vi "Same.vi"() -> ()   [LabVIEW 2017, in "Assertions.Tests.lvlib" / "Assert Not Equal.lvlib"]
uses:
  Assert Not Equal.lvlib
  src/Transparent Assertions/Constraints/IsEqual/IsEqual.lvclass
  C:/Users/pasca/Projects/Home/TransparentAssertions/src/Transparent Assertions/Constraints/Constraint/Constraint.lvclass
  src/Transparent Assertions/Constraints/IsEqual/Create.vi
  src/Transparent Assertions/Constraints/LogicalNot/LogicalNot.lvclass
  src/Transparent Assertions/Constraints/UnaryOperator/UnaryOperator.lvclass
  src/Transparent Assertions/Assertions/Assertions.lvlib
panel:
  out "error out":errorcluster
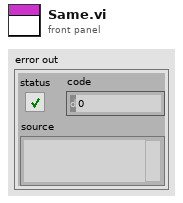
[diagram p1: front panel]
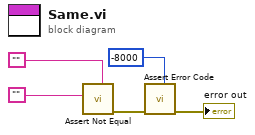
[diagram p0: block diagram]
diagram:
  n1 = call "Assert Not Equal.vi"("Expected"="", "Actual"="") -> ("error out"=w3:errorcluster)  [unwired: 9 in]
  n2 = call "Assert Error Code.vi"("Expected"=-8000, "error in (no error)"=w3) -> ("error out"=→"error out":errorcluster)  [unwired: 9 in]
